vi "1.vi"() -> ()   [LabVIEW 2018]
uses:
  <vilib>/measure/NI_MABase.lvlib
panel:
  in  "清零":bool
  in  "读取":bool
  in  "offset":dbl caption="偏移量" format="%0.2p"
  in  "phase":dbl caption="相位" format="%.2p"
  in  "amplitude":dbl=1.0 caption="幅值" format="%0.2p"
  in  "frequency":dbl=10.0 caption="频率" format="%0.2p"
  out "保存信息":string
  in  "数组":dbl[](array[numeric])
  in  "停止":bool
  in  "采集":bool
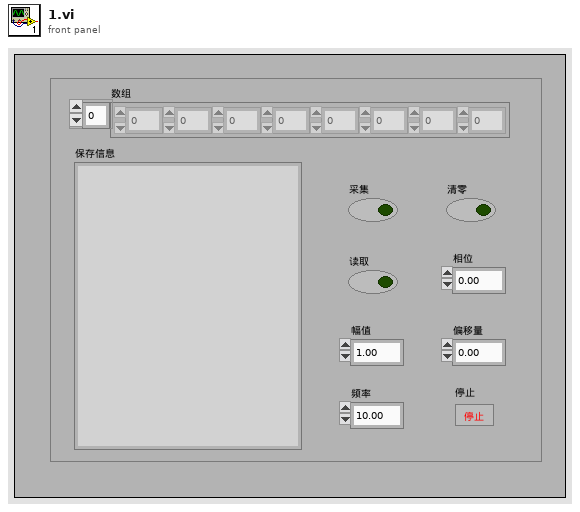
[diagram p1: front panel]
types:
  T1 = enum16{"open", "replace", "create", "open or create", "replace or create", "replace or create with confirmation"}
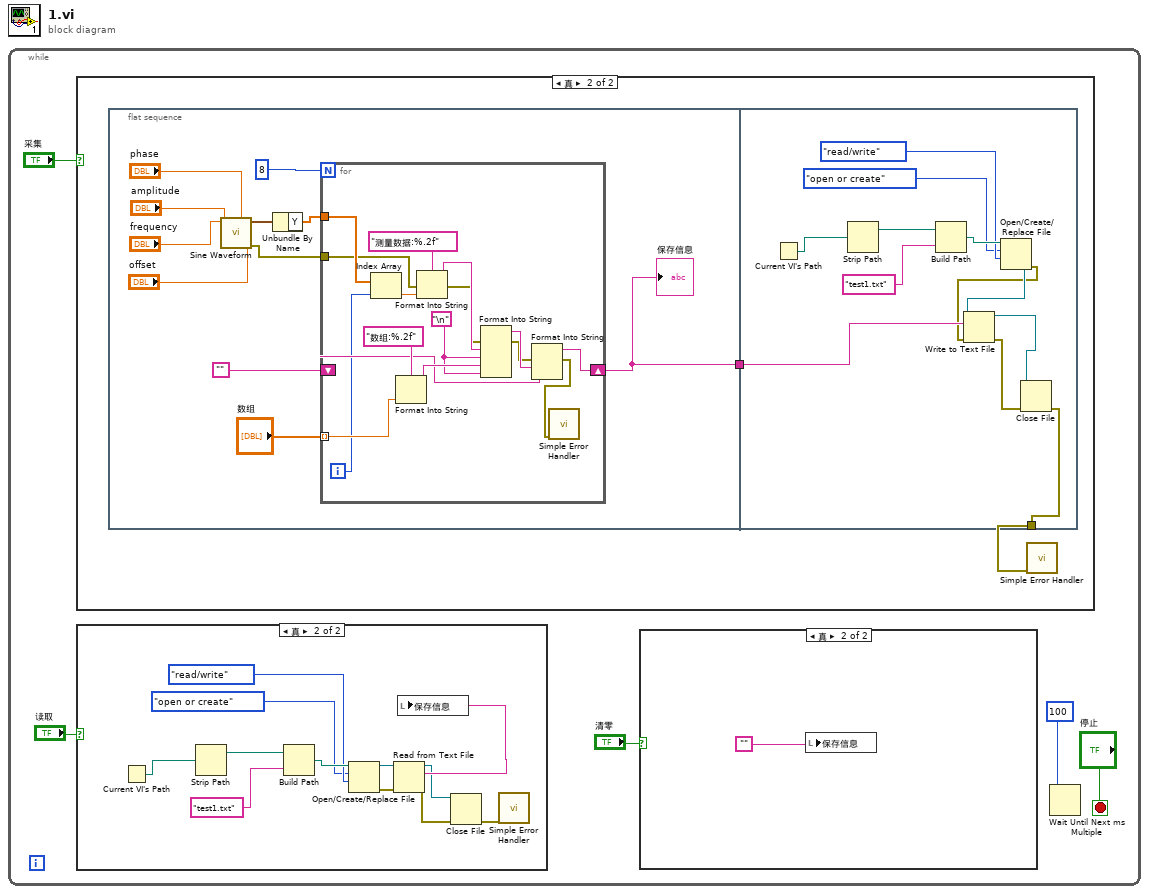
[diagram p0: block diagram]
diagram:
  n1 = while {
    stop <- "停止" stop-if-true
    n2 = case shown="真" "采集" {
      frame False {
      }
      frame True {
        n3 = flat-sequence {
          tunnel: [w22] -> w20
          tunnel: w20 -> [w53]
          tunnel: [w48] -> w19
          frame #0 {
            n4 = call <vilib>:"Sine Waveform.vi"("offset"="offset", "phase"="phase", "amplitude"="amplitude", "frequency"="frequency") -> ("error out"=w21:errorcluster, "signal out"=w26:waveform(dbl))  [unwired: 6 in]
            n5 = Unbundle By Name(w26) -> ("Y"=w25:dbl[])
            n6 = for {
              N: 8 -> [_]
              tunnel: "数组" -> [w44] mode=indexing
              shift-right: [w40] -> w22
              shift-left: "" -> [w39]
              tunnel: w25 -> [w38]
              tunnel: w21 -> [w35]
              i -> [w36]
              w45 = "\n"
              n7 = Index Array(array=w38, index=w36) -> (element=w37:dbl)
              n8 = Format Into String(format string="数组:%.2f" ("初始字符串"), w44) -> (resulting string=w46:string)  [unwired: 2 in, 1 out]
              n9 = Format Into String(format string="测量数据:%.2f" ("格式字符串"), error in=w35, w37) -> (resulting string=w42:string, error out=w34:errorcluster)  [unwired: 1 in]
              n10 = Format Into String(error in=w34, w42, w45, w46, w45) -> (resulting string=w41:string, error out=w33:errorcluster)  [unwired: 2 in]
              n11 = Format Into String(error in=w33, w41, w39) -> (resulting string=w40:string, error out=w32:errorcluster)  [unwired: 2 in]
              n12 = call <vilib>:"Simple Error Handler.vi"("error in (no error)"=w32) -> ()  [unwired: 4 in, 5 out]
            }
            "保存信息" <- w22
          }
          frame #1 {
            n13 = Current VI's Path() -> (path=w57:path)
            n14 = Strip Path(path=w57) -> (stripped path=w58:path)  [unwired: 1 out]
            n15 = Build Path(base path=w58, name or relative path="test1.txt") -> (appended path=w59:path)
            n16 = Open/Create/Replace File(file path (use dialog)=w59, operation (0:open)=T1."open or create" ("操作(0:open)"), access (0:read/write)=enum16{"read/write", "read-only", "write-only"}."read/write" ("权限(0:read/write)")) -> (refnum out=w52:refnum<file>, error out=w51:errorcluster)  [unwired: 3 in, 1 out]
            n17 = Write to Text File(file (use dialog)=w52, text=w53, error in=w51) -> (refnum out=w50:refnum<file>, error out=w49:errorcluster)  [unwired: 1 in, 1 out]
            n18 = Close File(refnum=w50, error in=w49) -> (error out=w48:errorcluster)  [unwired: 1 out]
          }
        }
        n19 = call <vilib>:"Simple Error Handler.vi"("error in (no error)"=w19) -> ()  [unwired: 4 in, 5 out]
      }
    }
    n20 = case shown="真" "读取" {
      frame False {
      }
      frame True {
        n21 = Current VI's Path() -> (path=w16:path)
        n22 = Strip Path(path=w16) -> (stripped path=w17:path)  [unwired: 1 out]
        n23 = Build Path(base path=w17, name or relative path="test1.txt") -> (appended path=w18:path)
        n24 = Open/Create/Replace File(file path (use dialog)=w18, operation (0:open)=T1."open or create" ("操作(0:open)"), access (0:read/write)=enum16{"read/write", "read-only", "write-only"}."read/write" ("权限(0:read/write)")) -> (refnum out=w12:refnum<file>, error out=w8:errorcluster)  [unwired: 3 in, 1 out]
        n25 = Read from Text File(file (use dialog)=w12, error in=w8) -> (refnum out=w10:refnum<file>, text=w11:string, error out=w9:errorcluster)  [unwired: 2 in, 1 out]
        n26 = local write "保存信息"(w11) -> ()
        n27 = Close File(refnum=w10, error in=w9) -> (error out=w7:errorcluster)  [unwired: 1 out]
        n28 = call <vilib>:"Simple Error Handler.vi"("error in (no error)"=w7) -> ()  [unwired: 4 in, 5 out]
      }
    }
    n29 = case shown="真" "清零" {
      frame False {
      }
      frame True {
        n30 = local write "保存信息"("") -> ()
      }
    }
    n31 = Wait Until Next ms Multiple(millisecond multiple=100) -> ()  [unwired: 1 out]
  }
